vi "PowerOff.vi"(0 "DashboardServer in":refnum<class "Dashboard Server.lvclass">, 5 "error in (no error)":errorcluster) -> (14 "DashboardServer out":refnum<class "Dashboard Server.lvclass">, 19 "error out":errorcluster)   [LabVIEW 2016, in "Dashboard Server.lvclass"]
uses:
  Dashboard Server.lvclass
panel:
  out "returnStatus":string
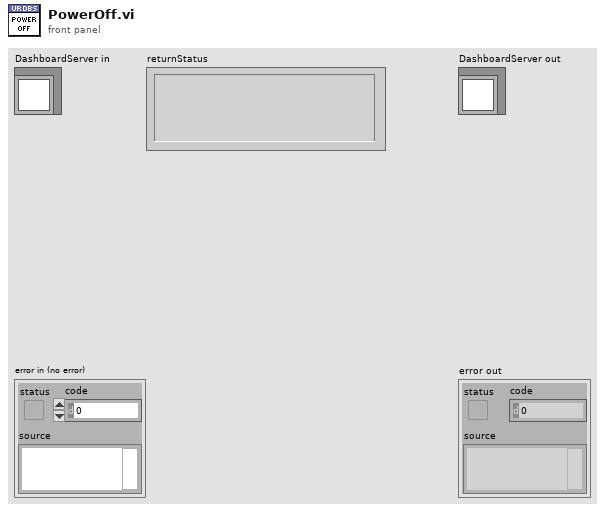
[diagram p1: front panel]
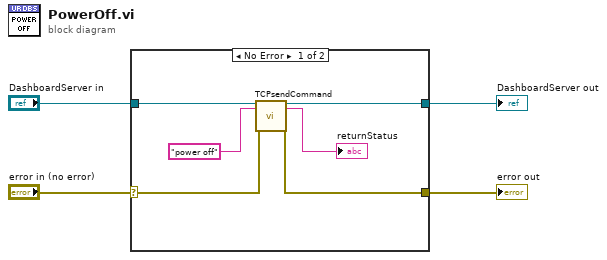
[diagram p0: block diagram]
diagram:
  n1 = case shown="No Error" "error in (no error)" {
    selector: "error in (no error)" -> [w8 w12]
    tunnel: [w7 w12] -> w3
    tunnel: [w9 w11] -> w1
    tunnel: "DashboardServer in" -> [w10 w11]
    frame No Error {
      n2 = call-dynamic "TCPsendCommand.vi"("DashboardServer in"=w10, "command"="power off", "error in (no error)"=w8) -> ("DashboardServer out"=w9:refnum<class "Dashboard Server.lvclass">, "returnStatus"=→"returnStatus":string, "error out"=w7:errorcluster)  [unwired: 13 in, 1 out]
    }
    frame Error {
    }
  }
  "error out" <- w3
  "DashboardServer out" <- w1
